vi "Get Config.vi"(8 "error in (no error)":errorcluster, 11 "DeployTcpResource in":refnum<class "TcpResource.lvclass">) -> (0 "error out":errorcluster, 2 "Config":T1[](array[typedef]), 3 "DeployTcpResource out":refnum<class "TcpResource.lvclass">)   [LabVIEW 2020, in "PicoG-Core.lvlib" / "TcpResource.lvclass"]
uses:
  TcpResource.lvclass
  TcpResource.lvclass/TcpResource.ctl
  Resource/Config Item.ctl
  Resource/Resource.lvclass
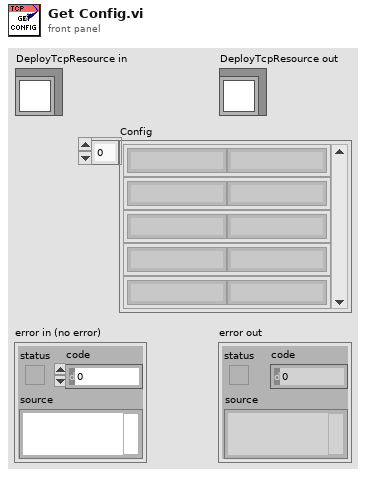
[diagram p1: front panel]
types:
  T1 = typedef "PicoG-Core.lvlib/Resource.lvclass/Config Item.ctl" = cluster{"Key":string, "Value":string}
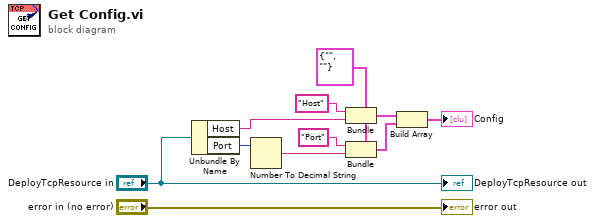
[diagram p0: block diagram]
diagram:
  w9 = T1 {"Key"="", "Value"=""} ("Config Item")
  n1 = Unbundle By Name("DeployTcpResource in") -> ("Host"=w6:string, "Port"=w10:u16)
  n2 = Number To Decimal String(number=w10) -> (decimal integer string=w8:string)  [unwired: 1 in]
  n3 = Bundle(cluster=w9, "Key"="Host", "Value"=w6) -> (w4:T1)
  n4 = Bundle(cluster=w9, "Key"="Port", "Value"=w8) -> (w3:T1)
  n5 = Build Array(w4, w3) -> (→"Config":T1[])
  "error out" <- "error in (no error)"
  "DeployTcpResource out" <- "DeployTcpResource in"
